vi "Initialize Attributes.vi"(8 "error in (no error)":errorcluster, 10 "Attribute Data":variant, 11 "IVI_PwrMeter in":refnum<class "IVI_PwrMeter.lvclass">) -> (0 "error out":errorcluster, 2 "Found?":bool, 3 "IVI_PwrMeter out":refnum<class "IVI_PwrMeter.lvclass">)   [LabVIEW 2013, in "IVI_PwrMeter.lvlib" / "IVI_PwrMeter.lvclass"]
doc: "Initialize object attribute.\n\nUnique resources should be allocated elsewhere!"
uses:
  IVI_PwrMeter.lvclass
  Core/Actors/CS++DeviceActor/CS++DeviceActor.lvclass
  IVI_PwrMeter.lvclass/IVI_PwrMeter.ctl
  Core/Libraries/Base/CS++Base.lvlib
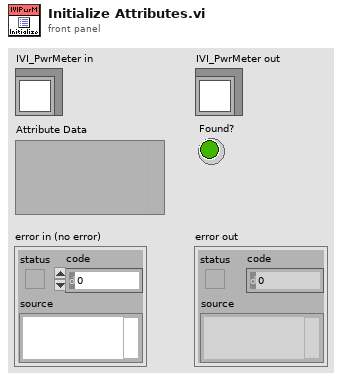
[diagram p1: front panel]
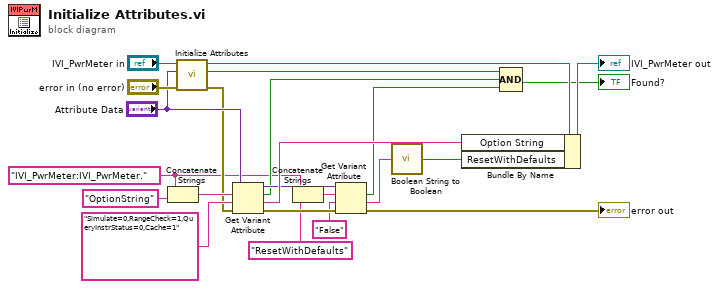
[diagram p0: block diagram]
diagram:
  w6 = "IVI_PwrMeter:IVI_PwrMeter."
  n1 = Concatenate Strings(w6, "OptionString" ("string")) -> (w20:string)
  n2 = call-parent "Initialize Attributes.vi"("error in (no error)"="error in (no error)", "Attribute Data"="Attribute Data", "CS++DeviceActor in"="IVI_PwrMeter in") -> ("error out"=w13:errorcluster, "Found?"=w14:bool, "CS++DeviceActor out"=w17:refnum<class "IVI_PwrMeter.lvclass">)  [unwired: 6 in]
  n3 = Get Variant Attribute(Variant="Attribute Data", name=w20, default value (empty Variant)="Simulate=0,RangeCheck=1,QueryInstrStatus=0,Cache=1" ("string"), error in=w13) -> (duplicate Variant=w10:variant, found=w8:bool, value=w15:string, error out=w12:errorcluster)
  n4 = Concatenate Strings(w6, "ResetWithDefaults" ("string")) -> (w7:string)
  n5 = Get Variant Attribute(Variant=w10, name=w7, default value (empty Variant)="False" ("string"), error in=w12) -> (found=w4:bool, value=w3:string, error out=→"error out":errorcluster)  [unwired: 1 out]
  n6 = call "Boolean String to Boolean.vi"("T/F String"=w3) -> ("Value"=w2:bool)
  n7 = Bundle By Name(cluster=w17, "Option String"=w15, "ResetWithDefaults"=w2) -> (→"IVI_PwrMeter out":refnum<class "IVI_PwrMeter.lvclass">)
  n8 = Compound Arithmetic op=AND(w14, w8, w4) -> (→"Found?":bool)
